vi "PostStepActions.vi"(8 "error in (no error)":errorcluster, 11 "TapeDrive in":refnum<class "TapeDrive.lvclass">) -> (0 "error out":errorcluster, 2 "maxVel":dbl[](array[numeric]), 3 "TapeDrive out":refnum<class "TapeDrive.lvclass">)   [LabVIEW 2020, in "TapeDrive.lvclass"]
uses:
  TapeDrive.lvclass
  TapeDrive.lvclass/TapeDrive.ctl
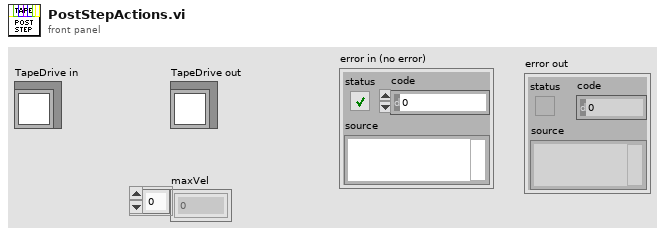
[diagram p1: front panel]
types:
  T1 = typedef "OnOffTypeDef.ctl" = enum16{"off", "on"}
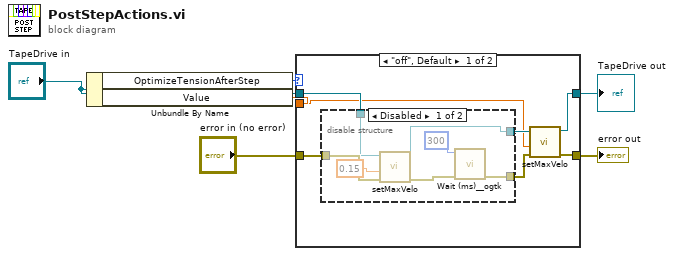
[diagram p0: block diagram]
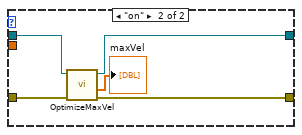
[diagram p3: hidden frame]
diagram:
  n1 = Unbundle By Name("TapeDrive in") -> ("OptimizeTensionAfterStep"=w5:T1, "Value"=w1:dbl)
  n2 = case shown="\"off\", Default" w5 {
    tunnel: "TapeDrive in" -> [w12 w27]
    tunnel: [w8 w26] -> w4
    tunnel: "error in (no error)" -> [w13 w25]
    tunnel: [w10 w24] -> w2
    tunnel: w1 -> [w7 _]
    frame "off", Default {
      n3 = disable-structure shown="Disabled" {
        disable-tunnel: w13 -> [w20 w21]
        disable-tunnel: w12 -> [w19 w22]
        disable-tunnel: [w17 w21] -> w11
        disable-tunnel: [w14 w22] -> w9
        frame Disabled {
          n4 = call "setMaxVelo.vi"("error in (no error)"=w20, "NewVal"=0.15, "TapeDrive in"=w19) -> ("error out"=w18:errorcluster, "TapeDrive out"=w14:refnum<class "TapeDrive.lvclass">)  [unwired: 6 in, 1 out]
          n5 = call "Wait (ms)__ogtk.vi"("error in (no error)"=w18, "milliseconds to wait"=u32 300) -> ("error out"=w17:errorcluster)  [unwired: 8 in, 1 out]
        }
        frame Enabled {
        }
      }
      n6 = call "setMaxVelo.vi"("error in (no error)"=w11, "NewVal"=w7, "TapeDrive in"=w9) -> ("error out"=w10:errorcluster, "TapeDrive out"=w8:refnum<class "TapeDrive.lvclass">)  [unwired: 6 in, 1 out]
    }
    frame "on" {
      n7 = call "OptimizeMaxVel.vi"("error in (no error)"=w25, "TapeDrive in"=w27) -> ("error out"=w24:errorcluster, "maxVel"=→"maxVel":dbl[], "TapeDrive out"=w26:refnum<class "TapeDrive.lvclass">)  [unwired: 7 in]
    }
  }
  "TapeDrive out" <- w4
  "error out" <- w2
